vi "gyro_test.vi"() -> ()   [LabVIEW 2021]
uses:
  <vilib>/myRIO/Instrument Drivers/Onboard IO/I2C/typedefs/I2C User Configuration.ctl
  <vilib>/myRIO/Instrument Drivers/Onboard IO/I2C/typedefs/I2C Transfer Rate.ctl
  <vilib>/Platform/TimedLoop/XDataNode/timing_clust.ctl
  <vilib>/Platform/TimedLoop/XDataNode/nitl_modes.ctl
  <vilib>/Platform/TimedLoop/XDataNode/wakeup.ctl
  <vilib>/myRIO/Instrument Drivers/Onboard IO/DIO/typedefs/DIO Reference.ctl
  <vilib>/myRIO/Common/Instrument Driver Framework/Utilities/typedefs/myRIO Generic Hardware Reference.ctl
  <vilib>/myRIO/Common/Instrument Driver Framework/Utilities/typedefs/Hardware Version Enum.ctl
  <vilib>/myRIO/Common/Instrument Driver Framework/Utilities/typedefs/myRIO v1.0 Reference.ctl
  <vilib>/myRIO/Common/Instrument Driver Framework/Utilities/typedefs/Generic FPGA Reference.ctl
  <vilib>/myRIO/Common/Instrument Driver Framework/myRIO v1.0/DIO/typedefs/DIO Channels List.ctl
  <vilib>/myRIO/Common/Instrument Driver Framework/myRIO v1.0/DIO/typedefs/DIO Channels Enum.ctl
  <vilib>/userDefined/High Color/nirio_resource_hc.ctl
  <vilib>/myRIO/Instrument Drivers/Onboard IO/I2C/typedefs/I2C Reference.ctl
  <vilib>/myRIO/Common/Instrument Driver Framework/myRIO v1.0/I2C/typedefs/I2C Channels Enum.ctl
  <vilib>/myRIO/Instrument Drivers/Onboard IO/I2C/typedefs/I2C Configuration.ctl
  <vilib>/myRIO/Common/Instrument Driver Framework/myRIO v1.0/DIO/vis/myRIO v1.1 Open DIO.vi
  <vilib>/myRIO/Common/Instrument Driver Framework/myRIO v1.0/I2C/vis/myRIO v1.1 Open I2C.vi
  <vilib>/myRIO/Common/Instrument Driver Framework/Utilities/vis/Validate Channels.vi
  <vilib>/myRIO/Common/Instrument Driver Framework/myRIO v1.0/DIO/vis/myRIO v1.0 Reserve DIO.vi
  <vilib>/myRIO/Common/Instrument Driver Framework/myRIO v1.0/I2C/vis/myRIO v1.0 Reserve I2C.vi
  <vilib>/myRIO/Common/Instrument Driver Framework/myRIO v1.0/UART/vis/myRIO v1.0 Close UART.vi
  <vilib>/myRIO/Common/Instrument Driver Framework/myRIO v1.0/Resource Manager/vis/myRIO v1.0 Reserve Channel List.vi
  <vilib>/myRIO/Common/Instrument Driver Framework/myRIO v1.0/DIO/vis/myRIO v1.0 Build MUX Configuration DIO.vi
  <vilib>/myRIO/Common/Instrument Driver Framework/myRIO v1.0/I2C/vis/myRIO v1.0 Build MUX Configuration I2C.vi
  <vilib>/myRIO/Common/Instrument Driver Framework/myRIO v1.0/Resource Manager/vis/myRIO v1.0 Reserve Channel.vi
  <vilib>/myRIO/Common/Instrument Driver Framework/myRIO v1.0/Resource Manager/vis/myRIO v1.0 Unreserve Channel.vi
  <vilib>/myRIO/Common/Instrument Driver Framework/myRIO v1.0/Resource Manager/vis/myRIO v1.0 Create Configuration List.vi
  <vilib>/myRIO/Common/Instrument Driver Framework/myRIO v1.0/Resource Manager/vis/myRIO v1.0 Build Mutex Name.vi
  <vilib>/Utility/VariantDataType/GetNumericInfo.vi
  <vilib>/Utility/error.llb/Error Cluster From Error Code.vi
  <vilib>/myRIO/Common/Instrument Driver Framework/myRIO v1.0/myRIO v1.1 Open.vi
  <vilib>/myRIO/Common/Instrument Driver Framework/Utilities/vis/IO Manager.vi
  <vilib>/myRIO/Common/Instrument Driver Framework/Utilities/vis/Configuration Manager.vi
  <vilib>/myRIO/Common/Instrument Driver Framework/myRIO v1.0/Resource Manager/vis/myRIO v1.0 Configure IO.vi
  <vilib>/myRIO/Common/Instrument Driver Framework/myRIO v1.0/myRIO v1.0 Close.vi
  <vilib>/myRIO/Common/Instrument Driver Framework/myRIO v1.0/I2C/vis/myRIO v1.0 Configure I2C.vi
  <vilib>/myRIO/Common/Instrument Driver Framework/myRIO v1.0/I2C/vis/myRIO v1.0 Write I2C.vi
  <vilib>/myRIO/Common/Instrument Driver Framework/myRIO v1.0/DIO/vis/myRIO v1.0 Read DIO.vi
  <vilib>/myRIO/Common/Instrument Driver Framework/myRIO v1.0/I2C/vis/myRIO v1.0 Read I2C.vi
  <vilib>/myRIO/Common/Instrument Driver Framework/myRIO v1.0/DIO/vis/myRIO v1.0 Write DIO.vi
  <vilib>/myRIO/Common/Instrument Driver Framework/Utilities/vis/FPGA Ref Manager.vi
  <vilib>/myRIO/Common/Instrument Driver Framework/myRIO v1.0/myRIO v1.0 Reset FPGA.vi
  <vilib>/myRIO/Common/Instrument Driver Framework/myRIO v1.0/IRQ/vis/myRIO v1.0 IRQ Info FGV.vi
  <vilib>/myRIO/Common/Instrument Driver Framework/myRIO v1.0/IRQ/vis/myRIO v1.0 Timer IRQ Info FGV.vi
  <vilib>/myRIO/Common/Instrument Driver Framework/myRIO v1.0/IRQ/vis/myRIO v1.0 ISR Agent.vi
  <vilib>/myRIO/Instrument Drivers/Utilities/vis/Reset Index.vi
  <vilib>/myRIO/Common/Instrument Driver Framework/myRIO v1.0/Resource Manager/vis/myRIO v1.0 Block Write Resource Manager.vi
  <vilib>/myRIO/Instrument Drivers/Onboard IO/I2C/vis/myRIO I2C Open.xnode
  <vilib>/myRIO/Instrument Drivers/Onboard IO/DIO/vis/myRIO DIO Open.xnode
  <vilib>/platform/TimedLoop/XDataNode/XDataNode.xnode
  <vilib>/myRIO/Instrument Drivers/Onboard IO/I2C/I2C.lvlib
  <vilib>/myRIO/Instrument Drivers/Onboard IO/DIO/DIO.lvlib
  <vilib>/Platform/TimedLoop/XDataNode/XDNodeRunTimeDep.lvlib
  <vilib>/myRIO/Instrument Drivers/Utilities/Utilities.lvlib
  <vilib>/ptbypt/NI_PtbyPt.lvlib
panel:
  out "output cluster":T1
  in  "OK Button":bool
  out "Bytes Read":u8[](array[numeric]) format="%x"
  out "X":i16
  out "Y":i16
  out "Z":i16
  out "angular rate":cluster{i16, i16, i16}(graph)
  in  "stop":bool
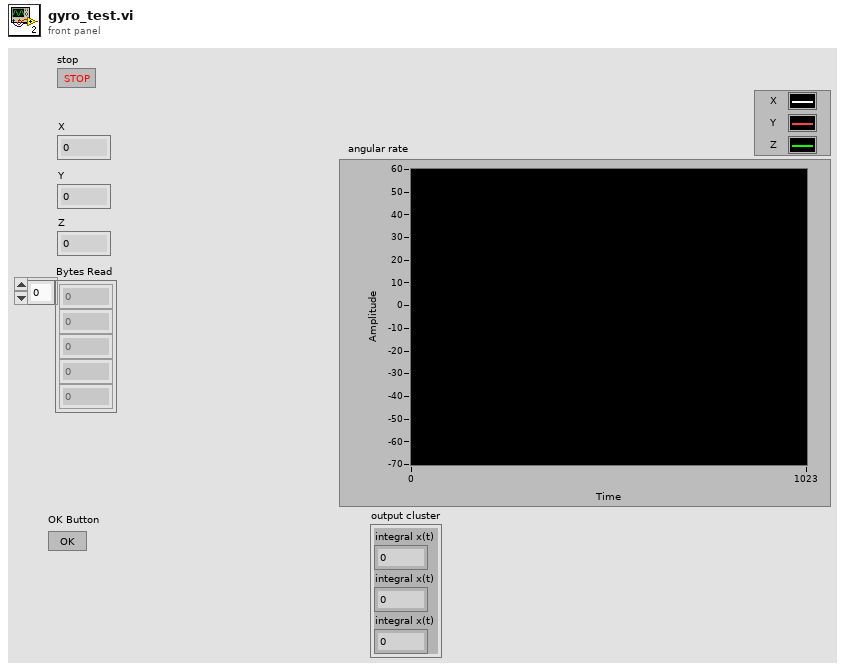
[diagram p1: front panel]
types:
  T1 = cluster{"integral x(t)":dbl, "integral x(t)":dbl, "integral x(t)":dbl}
  T2 = typedef "I2C.lvlib/I2C User Configuration.ctl" = cluster{"I2C Transfer Rate":T3}
  T3 = typedef "I2C.lvlib/I2C Transfer Rate.ctl" = enum16{"Standard mode (100 kbps)", "Fast mode (400 kbps)"}
  T4 = typedef "I2C.lvlib/I2C Reference.ctl" = cluster{"myRIO Reference":T5, "I2C Channels Enum":T9, "I2C Configuration":T10}
  T5 = typedef "myRIO Generic Hardware Reference.ctl" = cluster{"myRIO Model":T6, "myRIO Hardware Reference":T7}
  T6 = typedef "Hardware Version Enum.ctl" = enum16{"Unknown", "myRIO-1900", "myRIO-1950", "roboRIO", "NI ELVIS RIO CM", "ELVIS III"}
  T7 = typedef "myRIO v1.0 Reference.ctl" = cluster{"Generic FPGA Reference":T8, "Allow multiple opens":bool}
  T8 = typedef "Generic FPGA Reference.ctl" = refnum<k20>
  T9 = typedef "I2C Channels Enum.ctl" = enum16{"Not Connected", "A/I2C", "B/I2C", "I2C/I2C"}
  T10 = typedef "I2C.lvlib/I2C Configuration.ctl" = cluster{"I2C Transfer Rate":T3}
  T11 = typedef "DIO.lvlib/DIO Reference.ctl" = cluster{"myRIO Reference":T5, "DIO Channels List":T12}
  T12 = typedef "DIO Channels List.ctl" = T13[]
  T13 = typedef "DIO Channels Enum.ctl" = enum16{"Not Connected", "C/DIO0", "C/DIO1", "C/DIO2", "C/DIO3", "C/DIO4", "C/DIO5", "C/DIO6", "C/DIO7", "A/DIO0", "A/DIO1", "A/DIO2", "A/DIO3", "A/DIO4", "A/DIO5", "A/DIO6", "A/DIO7", "A/DIO8", "A/DIO9", "A/DIO10", "A/DIO11", "A/DIO12", "A/DIO13", "A/DIO14", "A/DIO15", "A/DIO16", "A/DIO17", "A/DIO18", "A/DIO19", "B/DIO0", "B/DIO1", "B/DIO2", "B/DIO3", "B/DIO4", "B/DIO5", "B/DIO6", "B/DIO7", "B/DIO8", "B/DIO9", "B/DIO10", "B/DIO11", "B/DIO12", "B/DIO13", "B/DIO14", "B/DIO15", "B/DIO16", "B/DIO17", "B/DIO18", "B/DIO19", "LED0", "LED1", "LED2", "LED3", "Button0", "DIO/DIO0", "DIO/DIO1", "DIO/DIO2", "DIO/DIO3", "DIO/DIO4", "DIO/DIO5", "DIO/DIO6", "DIO/DIO7", "DIO/DIO8", "DIO/DIO9", "SPI/CS0", "SPI/CS1", "SPI/CS2", "SPI/CS3", "LED RADIO (Green)", "LED RADIO (Red)", "LED COMM (Green)", "LED COMM (Red)", "LED MODE (Green)", "LED MODE (Red)"}
  T14 = typedef "XDNodeRunTimeDep.lvlib/timing_clust.ctl" = cluster{"Expected End [f-1]":u64, "Actual End [f-1]":u64, "Finished Late? [f-1]":bool, "Expected End [i-1]":u64, "Actual End [i-1]":u64, "Finished Late? [i-1]":bool, "Expected Start [i]":u64, "Actual Start [i]":u64, "Expected Start [f]":u64, "Actual Start [f]":u64, "Source Name":string, "Structure Name":string, "Period":i64, "Deadline":i64, "Offset":i64, "Start":i64, "Priority":i32, "Timeout":i32, "Mode":T15, "Wakeup Reason":T16, "Error":errorcluster, "Source Type":string, "Secondary Source Type":string, "Global End Time":u64, "Global Start Time":u64, "Frame Duration":u64, "Iteration Duration":u64, "Assigned CPU":i32, "I/O Scan Engine Mode":u32}
  T15 = typedef "XDNodeRunTimeDep.lvlib/nitl_modes.ctl" = enum32{"No Change", "Process missed periods, maintain original phase", "Discard missed periods, maintain original phase", "Process missed periods, ignore original phase", "Discard missed periods, ignore original phase"}
  T16 = typedef "XDNodeRunTimeDep.lvlib/wakeup.ctl" = enum32{"Normal", "Aborted", "Asynchronous wakeup", "Timing source error", "Timed loop error", "Timeout"}
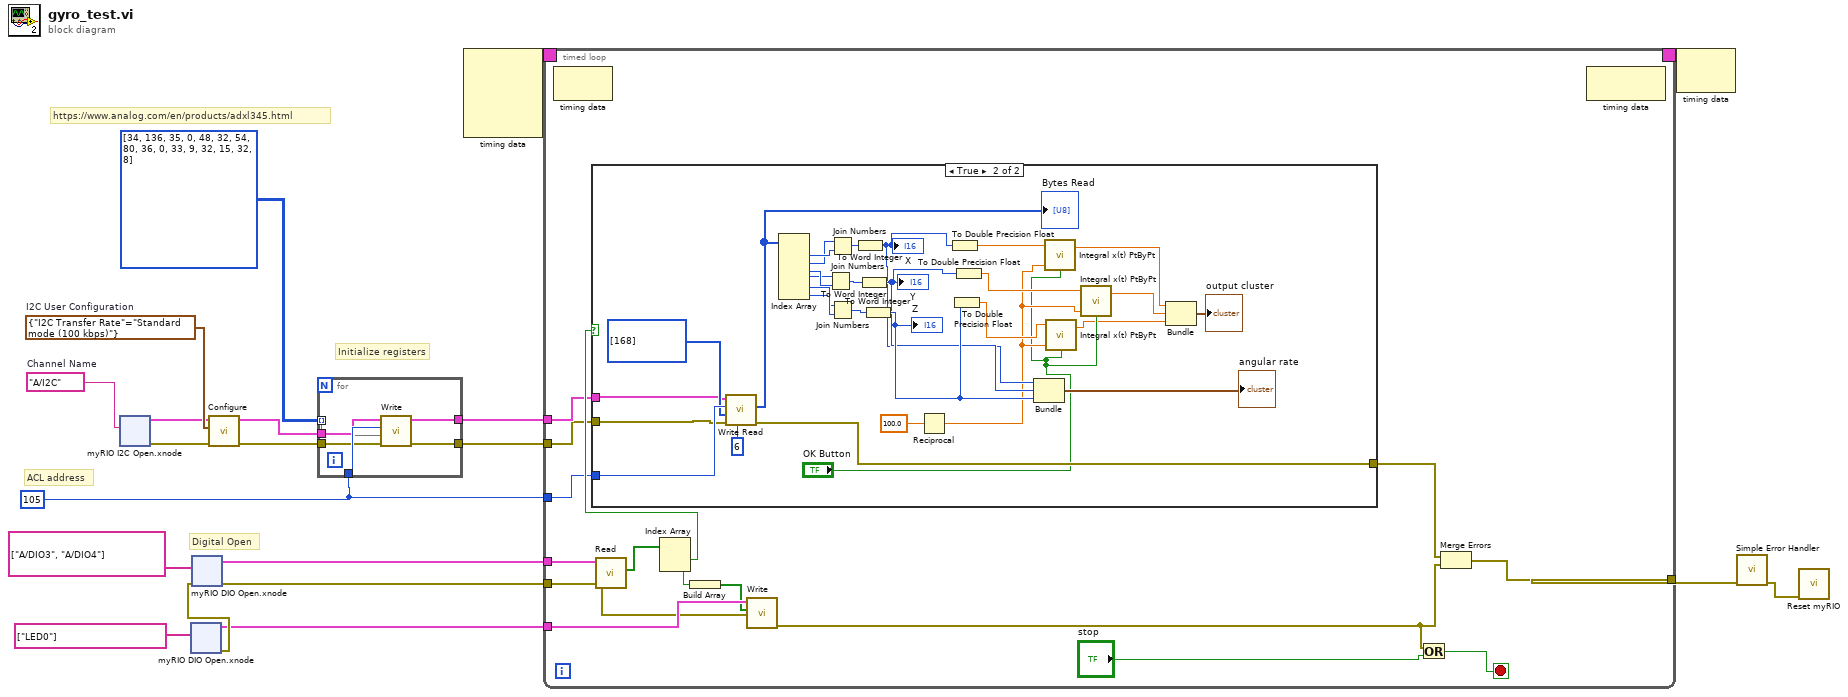
[diagram p0: block diagram]
diagram:
  w4 = u8 105 ("Slave Address (7-bit)")
  w17 = T2 {"I2C Transfer Rate"=enum."Standard mode (100 kbps)"}  # I2C User Configuration
  w18 = tag "A/I2C"  # Channel Name
  # "Digital Open"
  # "ACL address"
  # "https://www.analog.com/en/products/adxl345.html"
  # "Initialize registers"
  n1 = xnode "myRIO I2C Open.xnode"("Channel Name"=w18) -> ("error out"=w15:errorcluster, "I2C Ref Out"=w16:T4)  [unwired: 2 in]
  n2 = xnode "myRIO DIO Open.xnode"("Channel Names"=tag[] ["LED0"]) -> ("error out"=w9:errorcluster, "DIO Ref Out"=w7:T11)  [unwired: 2 in]
  n3 = xnode "myRIO DIO Open.xnode"("error in (no error)"=w9, "Channel Names"=tag[] ["A/DIO3", "A/DIO4"]) -> ("error out"=w6:errorcluster, "DIO Ref Out"=w8:T11)  [unwired: 1 in]
  n4 = call <vilib>:"Configure.vi"("error in (no error)"=w15, "I2C User Configuration"=w17, "I2C Ref In"=w16) -> ("error out"=w13:errorcluster, "I2C Ref Out"=w14:T4)  [unwired: 7 in]
  n5 = for {
    tunnel: w4 -> [w26]
    tunnel: w14 -> [w25]
    tunnel: w13 -> [w24]
    tunnel: i32[][] [[34, 136], [35, 0], [48, 32], [54, 80], [36, 0], [33, 9], [32, 15], [32, 8]] -> [w23] mode=indexing
    tunnel: [w22] -> w5
    tunnel: [w21] -> w3
    n6 = call <vilib>:"Write.vi"("error in (no error)"=w24, "Bytes to Write"=w23, "Slave Address (7-bit)"=w26, "I2C Ref In"=w25) -> ("error out"=w21:errorcluster, "I2C Ref Out"=w22:T4)  [unwired: 6 in]
  }
  n7 = node-c288() -> (w20:T14)  [unwired: 4 in]
  n8 = timed-loop {
    tunnel: w8 -> [w42]
    tunnel: w7 -> [w41]
    tunnel: w6 -> [w40]
    timing: w20 -> [_]
    timing-out: [_] -> w19
    tunnel: w5 -> [w34]
    tunnel: w4 -> [w33]
    tunnel: w3 -> [w32]
    tunnel: [w30] -> w2
    stop <- w29 stop-if-true
    n9 = node-c288() -> ()  [unwired: 1 in, 1 out]
    n10 = call <vilib>:"Read.vi"("error in (no error)"=w40, "DIO Ref In"=w42) -> ("error out"=w39:errorcluster, "Values"=w38:bool[])  [unwired: 7 in, 1 out]
    n11 = Index Array(array=w38) -> (element #1=w37:bool, element #2=w36:bool)  [unwired: 2 in]
    n12 = case shown="True" w37 {
      tunnel: w34 -> [_ w58]
      tunnel: w33 -> [_ w73]
      tunnel: w32 -> [w43 w59]
      tunnel: [w43 w60] -> w31
      frame False {
      }
      frame True {
        n13 = call <vilib>:"Write Read.vi"("Byte Count"=u32 6, "error in (no error)"=w59, "Bytes to Write"=u8[] [168], "Slave Address (7-bit)"=w73, "I2C Ref In"=w58) -> ("error out"=w60:errorcluster, "Bytes Read"=w70:u8[])  [unwired: 3 in, 1 out]
        "Bytes Read" <- w70
        n14 = Index Array(array=w70) -> (element #1=w69:u8, element #2=w68:u8, element #3=w66:u8, element #4=w65:u8, element #5=w64:u8, element #6=w63:u8)  [unwired: 6 in]
        n15 = Join Numbers(hi=w65, lo=w66) -> ((hi.lo)=w62:u16)
        n16 = Join Numbers(hi=w68, lo=w69) -> ((hi.lo)=w67:u16)
        n17 = Join Numbers(hi=w63, lo=w64) -> ((hi.lo)=w61:u16)
        n18 = To Word Integer(number=w67) -> (16bit integer=w54:i16)
        "X" <- w54
        n19 = To Word Integer(number=w62) -> (16bit integer=w55:i16)
        "Y" <- w55
        n20 = To Word Integer(number=w61) -> (16bit integer=w56:i16)
        "Z" <- w56
        n21 = Reciprocal(x=100.0) -> (1/x=w49:dbl)
        n22 = To Double Precision Float(number=w54) -> (double precision float=w52:dbl)
        n23 = To Double Precision Float(number=w56) -> (double precision float=w51:dbl)
        n24 = To Double Precision Float(number=w55) -> (double precision float=w50:dbl)
        n25 = Bundle(w54, w55, w56) -> (→"angular rate":cluster{i16, i16, i16})  [unwired: 1 in]
        n26 = call <vilib>:"Integral x(t) PtByPt.vi"("initialize"="OK Button", "dt"=w49, "x"=w52) -> ("integral x(t)"=w47:dbl)  [unwired: 1 in, 1 out]
        n27 = call <vilib>:"Integral x(t) PtByPt.vi"("initialize"="OK Button", "dt"=w49, "x"=w51) -> ("integral x(t)"=w45:dbl)  [unwired: 1 in, 1 out]
        n28 = call <vilib>:"Integral x(t) PtByPt.vi"("initialize"="OK Button", "dt"=w49, "x"=w50) -> ("integral x(t)"=w46:dbl)  [unwired: 1 in, 1 out]
        n29 = Bundle("integral x(t)"=w47, "integral x(t)"=w46, "integral x(t)"=w45) -> (→"output cluster":T1)  [unwired: 1 in]
      }
    }
    n30 = Build Array(w36) -> (w35:bool[])
    n31 = call <vilib>:"Write.vi"("error in (no error)"=w39, "Values"=w35, "DIO Ref In"=w41) -> ("error out"=w27:errorcluster)  [unwired: 6 in, 1 out]
    n32 = Or(x=w27, y="stop") -> (x .or. y?=w29:bool)
    n33 = Merge Errors(w31, w27) -> (w30:errorcluster)
    n34 = node-c288() -> ()  [unwired: 1 in, 1 out]
  }
  n35 = node-c288(w19) -> ()  [unwired: 1 out]
  n36 = call <vilib>:"Simple Error Handler.vi"("error in (no error)"=w2) -> ("error out"=w1:errorcluster)  [unwired: 4 in, 4 out]
  n37 = call <vilib>:"Reset myRIO.vi"("error in (no error)"=w1) -> ()  [unwired: 10 in, 1 out]
